vi "MB Ethernet Example Master MK2.vi"() -> ()   [LabVIEW 2021]
uses:
  API/Wrapper/API Main.lvlib
  API/Wrapper/Create TCP Master.vi
  API/Master/Modbus Master.lvclass
  Data Model/Identification Parameters.ctl
  Data Model/Device Data Model.lvclass
  Master Function Definition/Read Device ID code.ctl
panel:
  out "loop time":dbl
  in  "Read Device ID code":T1
  in  "Object ID":u8
  out "Objects":T2[](array[typedef]) {"Object ID" format="%x"}
  out "exception status":u8
  out "discrete inputs":bool[](array[boolean])
  out "Input Registers":u16[](array[numeric])=[0, 0, 2, 2]
  out "error out":errorcluster
  out "Holding Registers":u16[](array[numeric])=[0, 0, 2, 2]
  in  "Write Single Register":u16[](array[numeric])=[0, 0, 2, 2]
  in  "Write Multiple Registers":cluster{"Set Registers":bool, u16[]}={"Set Registers"=FALSE, [0, 0, 2, 2]}
  in  "Write Multiple Coils":T3={"Write Single Coils 2"=[TRUE, FALSE, FALSE, TRUE], "Set Coils"=FALSE}
  in  "Write Single Coils":bool[](array[boolean])=[FALSE, FALSE, FALSE, FALSE] caption="Coils to Write"
  in  "Address":string="localhost"
  in  "Stop":bool
  out "Coils":bool[](array[boolean])=[TRUE, FALSE, FALSE, TRUE] caption="Slave Discrete Inputs"
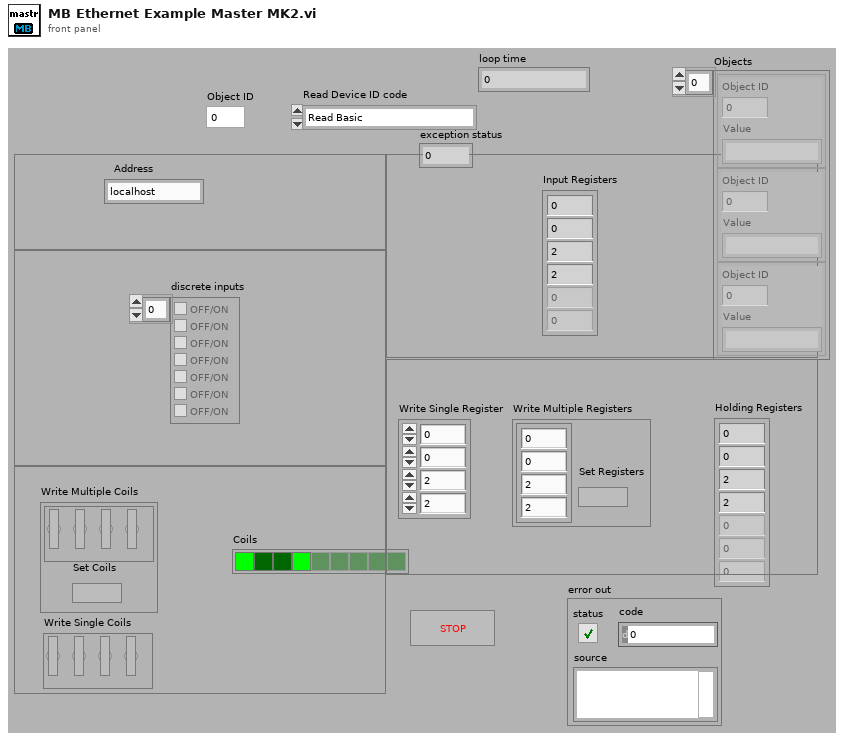
[diagram p1: front panel]
types:
  T1 = typedef "Device Data Model.lvclass/Read Device ID code.ctl" = enum8{"Read Basic", "Read Regular", "Read Extended", "Read Specific"}
  T2 = typedef "Device Data Model.lvclass/Identification Parameters.ctl" = cluster{"Object ID":u8, "Value":string}
  T3 = cluster{"Write Single Coils 2":bool[], "Set Coils":bool}
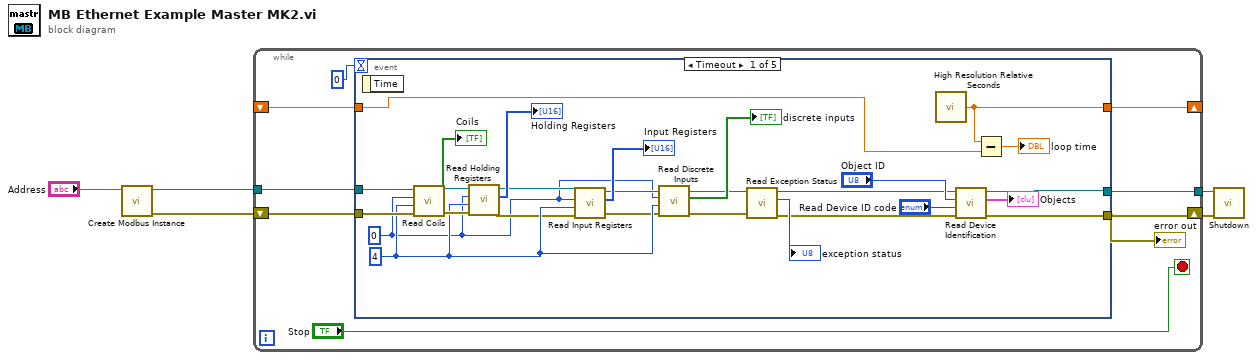
[diagram p0: block diagram]
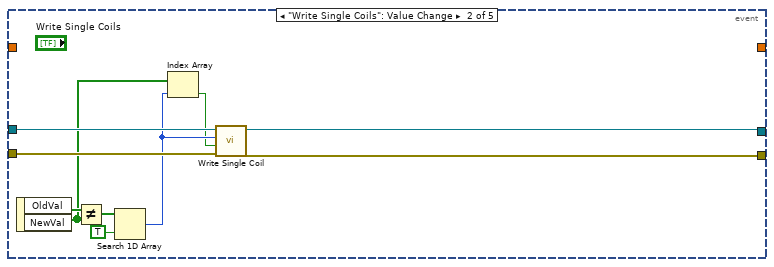
[diagram p2: hidden frame]
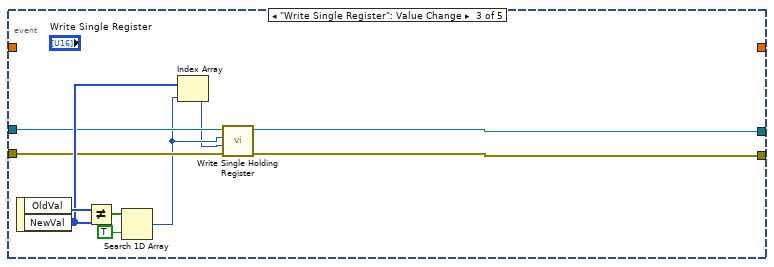
[diagram p3: hidden frame]
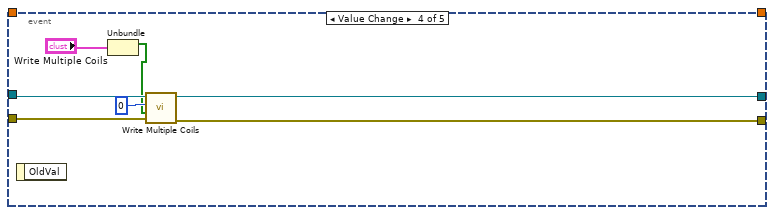
[diagram p4: hidden frame]
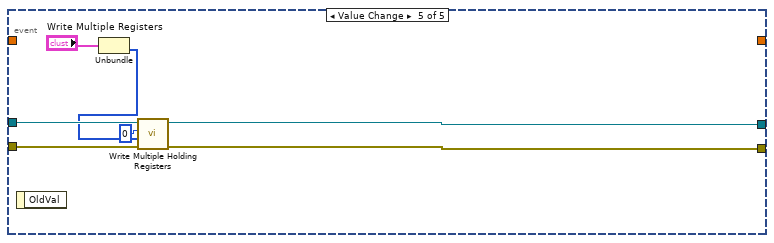
[diagram p5: hidden frame]
diagram:
  n1 = call-poly "Create Modbus Instance.vi"("address"="Address") -> ("error out"=w3:errorcluster, "TCP master instance"=w2:refnum<class "Modbus Master.lvclass">)  [unwired: 9 in]
  n2 = while {
    tunnel: w2 -> [w10]
    tunnel: [w9] -> w4
    shift-right: [w12] -> w5
    shift-left: w3 -> [w8]
    shift-right: [w7] -> _
    shift-left: _ -> [w6]
    stop <- "Stop" stop-if-true
    n3 = event shown="[0] Timeout" {
      selector: _ -> [_ _ _ _ _]
      dyn-events: _ -> [_ _ _ _ _]
      timeout: 0 -> [_ _ _ _ _]
      tunnel: [w17 w48 w56 w63 w70] -> w12
      tunnel: w10 -> [w40 w50 w54 w66 w72]
      tunnel: [w19 w47 w55 w62 w71] -> w9
      tunnel: w8 -> [w39 w49 w53 w65 w73]
      tunnel: [w16 _ _ _ _] -> w7
      tunnel: w6 -> [w15 _ _ _ _]
      event Timeout {
        w33 = u16 4 ("Number of coils")
        w26 = u16 0 ("Starting Address")
        n4 = event-data() -> ()  [unwired: 2 out]
        n5 = call-dynamic "Read Coils.vi"("error in (no error)"=w39, "number of coils"=w33, "starting address"=w26, "Modbus master in"=w40) -> ("error out"=w36:errorcluster, "coil values"=→"Coils":bool[], "Modbus master out"=w37:refnum<class "Modbus Master.lvclass">)  [unwired: 5 in]
        n6 = call-dynamic "Read Holding Registers.vi"("error in (no error)"=w36, "number of holding registers"=w33, "starting address"=w26, "Modbus master in"=w37) -> ("error out"=w29:errorcluster, "register values"=→"Holding Registers":u16[], "Modbus master out"=w30:refnum<class "Modbus Master.lvclass">)  [unwired: 5 in]
        n7 = call-dynamic "Read Input Registers.vi"("error in (no error)"=w29, "number of input registers"=w33, "starting address"=w26, "Modbus master in"=w30) -> ("error out"=w27:errorcluster, "register values"=→"Input Registers":u16[], "Modbus master out"=w28:refnum<class "Modbus Master.lvclass">)  [unwired: 5 in]
        n8 = call-dynamic "Read Discrete Inputs.vi"("error in (no error)"=w27, "number of discrete inputs"=w33, "starting address"=w26, "Modbus master in"=w28) -> ("error out"=w24:errorcluster, "discrete input values"=→"discrete inputs":bool[], "Modbus master out"=w25:refnum<class "Modbus Master.lvclass">)  [unwired: 5 in]
        n9 = call-dynamic "Read Exception Status.vi"("error in (no error)"=w24, "Modbus master in"=w25) -> ("error out"=w18:errorcluster, "exception status"=→"exception status":u8, "Modbus master out"=w20:refnum<class "Modbus Master.lvclass">)  [unwired: 7 in]
        n10 = call <vilib>:"High Resolution Relative Seconds.vi"() -> ("relative seconds"=w16:dbl)
        n11 = call-dynamic "Read Device Identification.vi"("error in (no error)"=w18, "read device ID code"="Read Device ID code", "object ID"="Object ID", "Modbus master in"=w20) -> ("error out"=w17:errorcluster, "objects"=→"Objects":cluster{"object ID":u8, "value":string}[], "Modbus master out"=w19:refnum<class "Modbus Master.lvclass">)  [unwired: 5 in]
        n12 = Subtract(x=w16, y=w15) -> (x-y=→"loop time":dbl)
      }
      event "Write Single Coils": Value Change {
        n13 = event-data() -> ("OldVal"=w46:bool[], "NewVal"=w43:bool[])  [unwired: 1 out]
        n14 = Not Equal?(x=w46, y=w43) -> (x != y?=w45:bool[])
        n15 = Search 1D Array(1D array=w45, element=TRUE) -> (index of element=w42:i32)  [unwired: 1 in]
        n16 = Index Array(array=w43, index=w42) -> (element=w41:bool)
        n17 = call-dynamic "Write Single Coil.vi"("error in (no error)"=w49, "coil value"=w41, "address"=w42, "Modbus master in"=w50) -> ("error out"=w48:errorcluster, "Modbus master out"=w47:refnum<class "Modbus Master.lvclass">)  [unwired: 6 in]
      }
      event "Write Single Register": Value Change {
        n18 = event-data() -> ("OldVal"=w58:u16[], "NewVal"=w57:u16[])  [unwired: 1 out]
        n19 = Not Equal?(x=w58, y=w57) -> (x != y?=w60:bool[])
        n20 = Search 1D Array(1D array=w60, element=TRUE) -> (index of element=w52:i32)  [unwired: 1 in]
        n21 = Index Array(array=w57, index=w52) -> (element=w51:u16)
        n22 = call-dynamic "Write Single Holding Register.vi"("error in (no error)"=w53, "holding register value"=w51, "address"=w52, "Modbus master in"=w54) -> ("error out"=w56:errorcluster, "Modbus master out"=w55:refnum<class "Modbus Master.lvclass">)  [unwired: 6 in]
      }
      event "Write Multiple Coils.Set Coils": Value Change {
        n23 = event-data() -> ()  [unwired: 2 out]
        n24 = Unbundle("Write Multiple Coils") -> ("Write Single Coils 2"=w61:bool[])  [unwired: 1 out]
        n25 = call-dynamic "Write Multiple Coils.vi"("error in (no error)"=w65, "coil values"=w61, "starting address"=u16 0 ("Starting Address"), "Modbus master in"=w66) -> ("error out"=w63:errorcluster, "Modbus master out"=w62:refnum<class "Modbus Master.lvclass">)  [unwired: 6 in]
      }
      event "Write Multiple Registers.Set Registers": Value Change {
        n26 = event-data() -> ()  [unwired: 2 out]
        n27 = Unbundle("Write Multiple Registers") -> (w68:u16[])  [unwired: 1 out]
        n28 = call-dynamic "Write Multiple Holding Registers.vi"("error in (no error)"=w73, "holding register values"=w68, "starting address"=u16 0 ("Starting Address"), "Modbus master in"=w72) -> ("error out"=w70:errorcluster, "Modbus master out"=w71:refnum<class "Modbus Master.lvclass">)  [unwired: 6 in]
      }
    }
    "error out" <- w12
  }
  n29 = call-dynamic "Shutdown.vi"("error in (no error)"=w5, "Modbus master in"=w4) -> ()  [unwired: 9 in, 1 out]
